vi "Auto Intake Mode.vi"(11 "Intake Commands Cluster":T2={"Intake Commands"=enum."Load", "Intake Mode"=enum."Auto", "Override IR"=FALSE}) -> (0 "Intake States":T1, 1 "Raw Negated Encoder Position":dbl, 2 "Roller Power":dbl, 3 "Angle Power":dbl, 4 "Target Height":dbl, 5 "Encoder Position":dbl, 6 "Rollers Active?":bool)   [LabVIEW 2015]
uses:
  Common Code/Intake Commands Cluster.ctl
  Common Code/Intake Commands.ctl
  Common Code/Intake Mode.ctl
  Common Code/Intake States.ctl
  Robot Global Data.vi
  <vilib>/addons/control/pid/pid.llb/PID (DBL).vi
  <vilib>/addons/control/pid/NI_PID_pid.lvlib
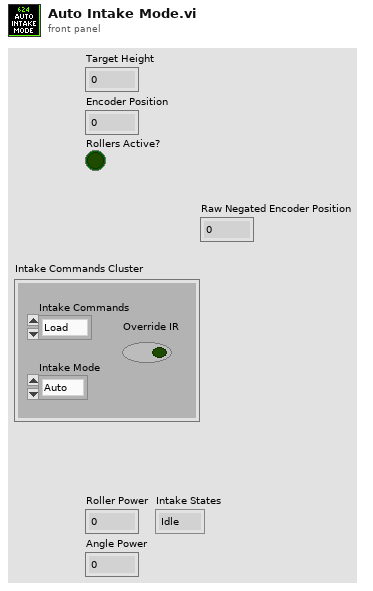
[diagram p1: front panel]
types:
  T1 = typedef "Intake States.ctl" = enum16{"Idle", "Set roller speed", "Move to angle"}
  T2 = typedef "Intake Commands Cluster.ctl" = cluster{"Intake Commands":T3, "Intake Mode":T4, "Override IR":bool}
  T3 = typedef "Intake Commands.ctl" = enum16{"Unload", "Load", "Pull up", "Drop low", "Idle", "Lift Half"}
  T4 = typedef "Intake Mode.ctl" = enum16{"Safe", "Auto", "Manual"}
  T5 = typedef "Dashboard Control Data.ctl" = cluster{"Encoder Control":T6, "Steer PID output":cluster{"output high":dbl, "output low":dbl}, " Steer PID gains":cluster{"proportional gain (Kc)":dbl, "integral time (Ti, min)":dbl, "derivative time (Td, min)":dbl}, "Drivetrain Settings":T7, "Vision Packet":T8, "Info/Command Cluster":T9, "Ball Vision Packet":T10, "Intake Presets":T12, "Intake Encoder Control":T14, "Climb Presets":T15, "Goal Output Range":cluster{"output high":dbl, "output low":dbl}, "Shooter Presets":T16}
  T6 = typedef "Encoder Control.ctl" = cluster{"Right Tick Constant":dbl, "Left Tick Constant":dbl, "Reset?":bool, "Y Dist":cluster{"PID gains":cluster{"proportional gain (Kc)":dbl, "integral time (Ti, min)":dbl, "derivative time (Td, min)":dbl}}, "Y Stop Thresh":dbl, "Y Stop Speed":dbl}
  T7 = typedef "Drivetrain Settings.ctl" = cluster{"Gyro Tolerance":dbl, "Throttle Ramp (ms)":dbl, "Angular rate compensation":bool, "Throttle to Rate Scale":dbl, "Rate compensation gain":dbl, "Kv":dbl, "Ka":dbl, "Feed Forward P":dbl, "Feed Forward D":dbl, "Goal Vision PID gains":cluster{"proportional gain (Kc)":dbl, "integral time (Ti, min)":dbl, "derivative time (Td, min)":dbl}, "Goal Detection Window":dbl}
  T8 = typedef "Goal Vision Packet.ctl" = cluster{"Distance":dbl, "Center X":dbl, "Center Y":dbl, "Found Target?":bool}
  T9 = typedef "Ball Tracking Command Cluster.ctl" = cluster{"Distance to Ball":dbl, "Desired Angle":dbl, "Command":enum16{"Turn to Ball", "Turn to Angle", "Get Distance"}, "Pixels from Center":dbl}
  T10 = typedef "Ball Vision Packet.ctl" = cluster{"Ball Detected?":bool, "Distance to Ball":dbl, "Desired Angle":dbl, "Pixels from Center":dbl, "Tracking mode":T11}
  T11 = typedef "Tracking Mode.ctl" = enum16{"Turn to Ball", "Turn to Angle"}
  T12 = typedef "Intake Presets.ctl" = cluster{"Intake Speed":dbl, "Outake Speed":dbl, "Low Height":dbl, "Half Height":dbl, "Full Height":dbl, "Angle Speed":dbl, "Fast Angle":dbl, "Encoder Scale":dbl, "Load Height":dbl, "Output Range":T13, "Rotation Power Max/Min":dbl, "MaxCurrent":dbl, "Intake Trip Time":dbl, "Idle Height":dbl, "Max Height":dbl, "Reset Encoders?":bool, "PID gains":cluster{"proportional gain (Kc)":dbl, "integral time (Ti, min)":dbl, "derivative time (Td, min)":dbl}}
  T13 = typedef "Drivetrain Output Range.ctl" = cluster{"output high":dbl, "output low":dbl}
  T14 = typedef "IntakeEcoderControl.ctl" = cluster{"Arm Tick Constant":dbl, "Reset?":bool, "Y Dist":cluster{"PID gains":cluster{"proportional gain (Kc)":dbl, "integral time (Ti, min)":dbl, "derivative time (Td, min)":dbl}}, "Y Stop Thresh":dbl, "Y Stop Speed":dbl}
  T15 = typedef "Climb Presets.ctl" = cluster{"Pull Power":dbl, "Unpin Power":dbl, "Time to Hold":dbl}
  T16 = typedef "Shooter Presets.ctl" = cluster{"Batter Shot":T17, "Deep Middle Shot":T17, "Manual Shot":T17, "Left Ticks Per Rotation":dbl, "Right Ticks Per Rotation":dbl, "Low Bar Shot":T17, "Shooter RPM Tolerance":dbl, "IIR Filter Power":dbl, "Trigger Power":dbl, "Fire from Load Delay":i32, "Angle Pot M":dbl, "Angle Pot B":dbl, "Shooter Length":dbl, "String Pot Dist":dbl, "Angle PID gains":cluster{"proportional gain (Kc)":dbl, "integral time (Ti, min)":dbl, "derivative time (Td, min)":dbl}, "Angle Motor Output":cluster{"output high":dbl, "output low":dbl}, "Shooter Angle Tolerance":dbl, "Vision Shoot x^2":dbl, "Vision Shoot x":dbl, "Dist from Axis Cam to Pivot":dbl, "High Goal Center Height":dbl, "Feed Forward Max Accel":dbl, "Feed Forward Kv":dbl, "Backwards Trigger":dbl, "Shot Finish Delay (ms)":dbl, "Angle Max Current":dbl, "Angle Current Trip Time":dbl, "Shooter Intake Angle":dbl, "Vision Shoot c":dbl, "Reset?":bool, "Servo Release Delay":dbl, "Servo Idle Angle":i32, "Servo Hold Angle":i32, "Angle Pot x^2":dbl, "Angle Pot x":dbl, "Angle Pot c":dbl}
  T17 = typedef "Shot Presets.ctl" = cluster{"Left Wheel RPM":dbl, "Right Wheel RPM":dbl, "Angle":dbl}
  T18 = cluster{"proportional gain (Kc)":dbl, "integral time (Ti, min)":dbl, "derivative time (Td, min)":dbl}
  T19 = typedef "WPI_MotorControlDeviceRef.ctl" = cluster{"DeviceStatus":errorcluster, "Type":T20, "PWM":cluster{"PWM Channel":T21, "DeadBand":T22}, "CAN":cluster{"Device Number":u8, "Control Mode":T23, "Semaphore":T24, "Max Vout":dbl, "TalonSRX Control Mode":T25}, "Invert":bool}
  T20 = typedef "WPI_MotorControlType.ctl" = enum16{"PWM", "CAN", "CANTalonSRX"}
  T21 = typedef "FPGA_DIOPWMChannel.ctl" = enum8{"PWM 0", "PWM 1", "PWM 2", "PWM 3", "PWM 4", "PWM 5", "PWM 6", "PWM 7", "PWM 8", "PWM 9", "PWM MXP 0", "PWM MXP 1", "PWM MXP 2", "PWM MXP 3", "PWM MXP 4", "PWM MXP 5", "PWM MXP 6", "PWM MXP 7", "PWM MXP 8", "PWM MXP 9", "Invalid"}
  T22 = typedef "WPI_PWMDeadband.ctl" = cluster{"Name":string, "maxPositivePwm":i32, "minPositivePwm":i32, "centerPwm":i32, "maxNegativePwm":i32, "minNegativePwm":i32, "angularRange":u16}
  T23 = typedef "WPI_CANJaguar_ControlMode.ctl" = enum8{"Percent VBus", "Current", "Speed", "Position", "Voltage"}
  T24 = typedef "Semaphore RefNum" = refnum<k1>
  T25 = typedef "WPI_CANTalonSRX_APIControlMode.ctl" = enum8{"Percent VBus", "Speed", "Position", "Slave", "Unchanged / Invalid", "Voltage Compensation", "Current", "Motion Profile"}
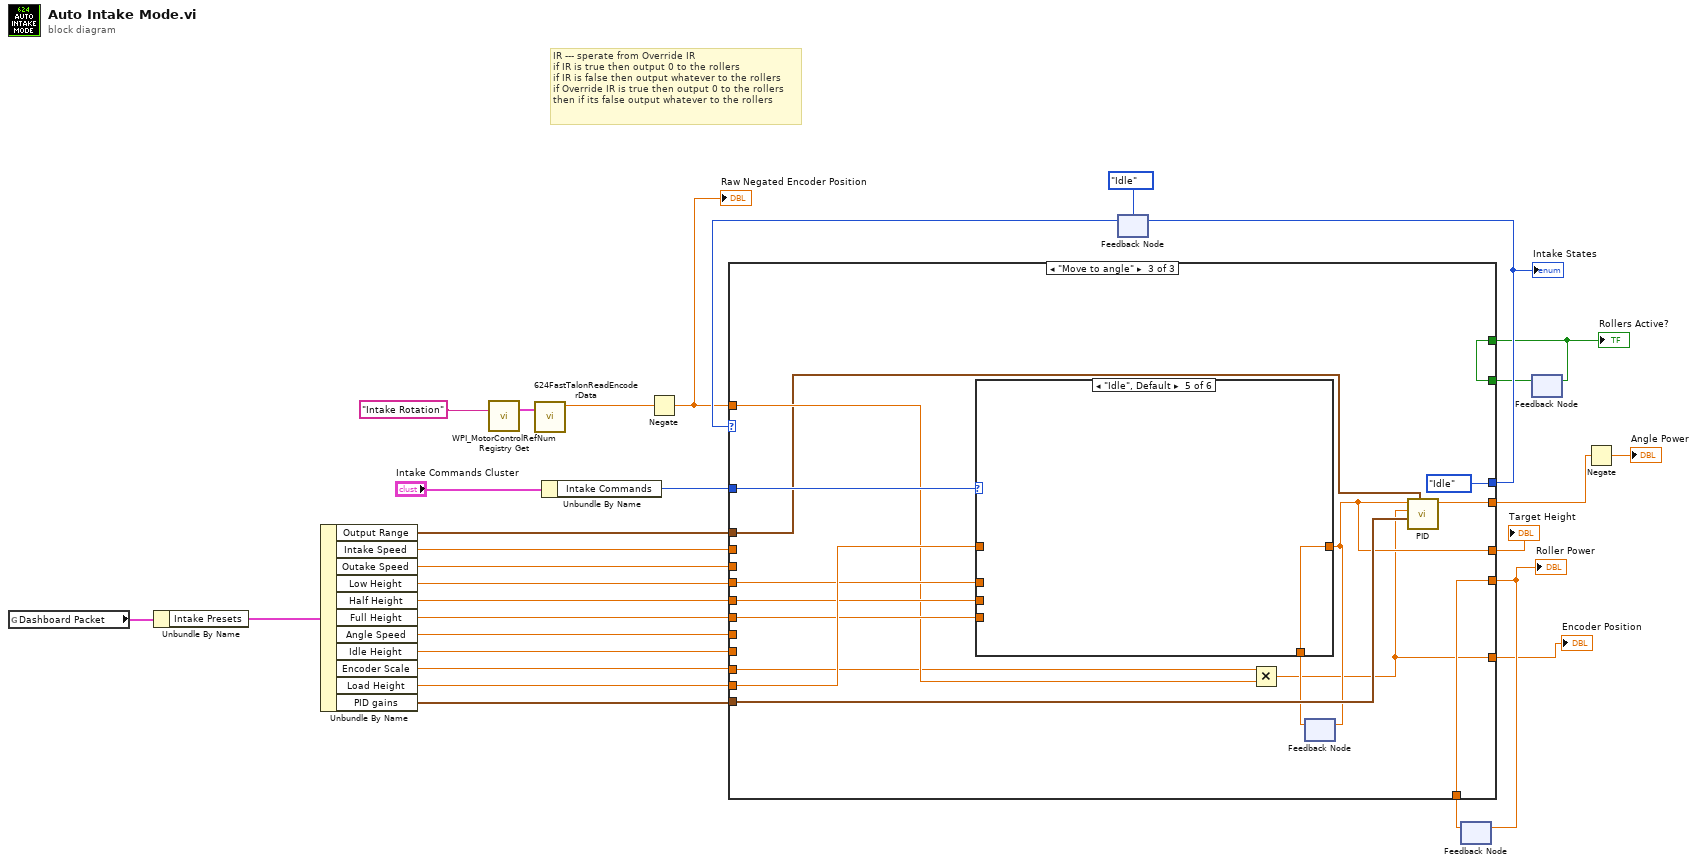
[diagram p0: block diagram]
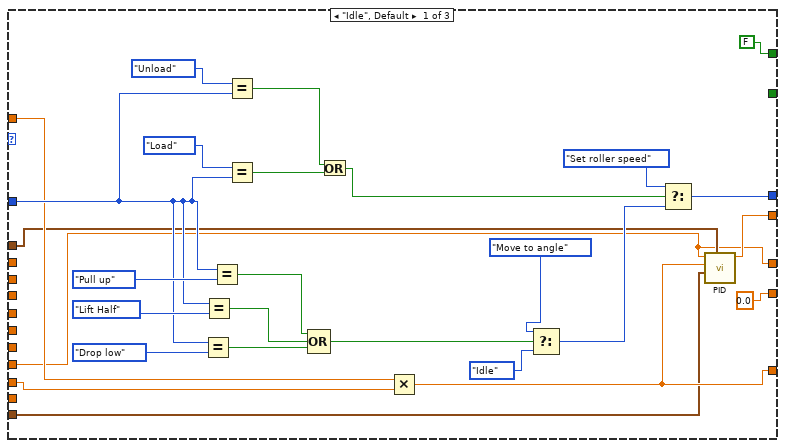
[diagram p2: hidden frame]
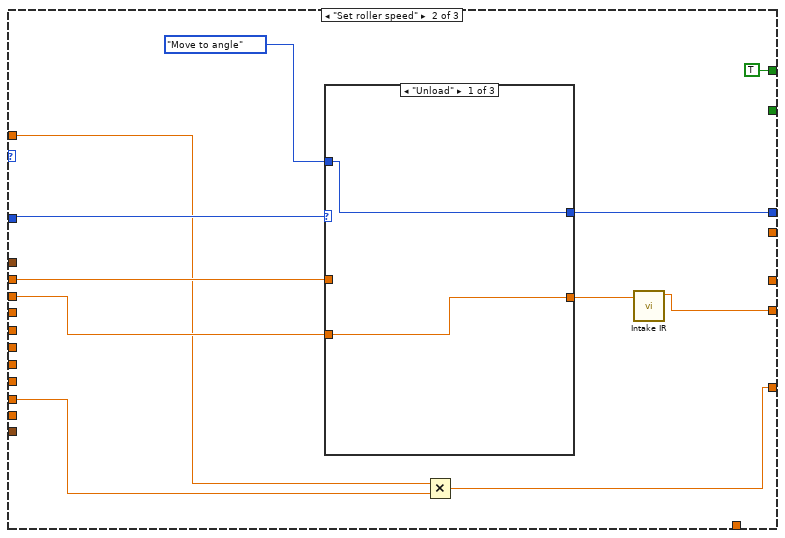
[diagram p3: hidden frame]
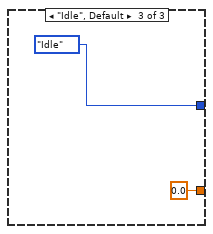
[diagram p5: hidden frame]
diagram:
  # "IR --- sperate from Override IR \nif IR is true then output 0 to the rollers\nif IR is false then output whatever to the rollers\nif Override IR is true then output 0 to the rollers\nthen if its false output whatever to the rollers"
  n1 = global read "Robot Global Data.vi" "Dashboard Packet"() -> (w1:T5)
  n2 = Unbundle By Name(w1) -> ("Intake Presets"=w2:T12)
  n3 = Unbundle By Name(w2) -> ("Output Range"=w13:T13, "Intake Speed"=w12:dbl, "Outake Speed"=w11:dbl, "Low Height"=w10:dbl, "Half Height"=w9:dbl, "Full Height"=w8:dbl, "Angle Speed"=w7:dbl, "Idle Height"=w6:dbl, "Encoder Scale"=w5:dbl, "Load Height"=w4:dbl, "PID gains"=w3:T18)
  n4 = call <vilib>:"WPI_MotorControlRefNum Registry Get.vi"("refnum name"="Intake Rotation") -> ("MotorControlDevRef"=w22:T19)  [unwired: 9 in, 1 out]
  n5 = call "624FastTalonReadEncoderData.vi"("CAN Talon SRX Ref"=w22) -> ("Encoder Position"=w19:dbl)  [unwired: 5 in, 5 out]
  n6 = Unbundle By Name("Intake Commands Cluster") -> ("Intake Commands"=w27:T3)
  n7 = Negate(x=w19) -> (-x=w18:dbl)
  "Raw Negated Encoder Position" <- w18
  n8 = feedback #1(Intake_States."Idle") -> (w29:T1)
  n9 = feedback #2() -> (w24:dbl)  [unwired: 1 in]
  n10 = feedback #3() -> (w16:bool)  [unwired: 1 in]
  n11 = case shown="\"Move to angle\"" w29 {
    tunnel: w27 -> [w43 w68 w90]
    tunnel: [w47 w66 Intake_States."Idle"] -> w26
    tunnel: w13 -> [w34 _ w79]
    tunnel: w11 -> [_ w64 _]
    tunnel: w8 -> [_ _ w85]
    tunnel: w12 -> [_ w65 _]
    tunnel: w9 -> [_ _ w87]
    tunnel: w7 -> [_ _ _]
    tunnel: w10 -> [_ _ w86]
    tunnel: [0.0 ("Intake Speed") w59 w89] -> w25
    tunnel: w24 -> [_ _ w89]
    tunnel: w4 -> [_ _ w88]
    tunnel: [w33 _ w83] -> w14
    tunnel: w18 -> [w37 w63 w82]
    tunnel: w5 -> [w38 w62 w81]
    tunnel: w3 -> [w35 _ w80]
    tunnel: w6 -> [w32 _ _]
    tunnel: [w32 _ w78] -> w21
    tunnel: [w36 w61 w76] -> w20
    tunnel: [FALSE TRUE w75] -> w17
    tunnel: w16 -> [_ _ w75]
    frame "Idle", Default {
      n12 = Equal?(x=w43, y=Intake_Commands."Drop low" ("Intake Commands")) -> (x = y?=w49:bool)
      n13 = Equal?(x=w43, y=Intake_Commands."Lift Half" ("Intake Commands")) -> (x = y?=w50:bool)
      n14 = Equal?(x=w43, y=Intake_Commands."Pull up" ("Intake Commands")) -> (x = y?=w54:bool)
      n15 = Equal?(x=Intake_Commands."Unload" ("Intake Commands"), y=w43) -> (x = y?=w42:bool)
      n16 = Equal?(x=Intake_Commands."Load" ("Intake Commands"), y=w43) -> (x = y?=w41:bool)
      n17 = Compound Arithmetic op=OR(w54, w50, w49) -> (w53:bool)
      n18 = Or(x=w42, y=w41) -> (x .or. y?=w40:bool)
      n19 = Multiply(x=w37, y=w38) -> (x*y=w36:dbl)
      n20 = Select(t=Intake_States."Move to angle", s=w53, f=Intake_States."Idle") -> (s? t:f=w48:T1)
      n21 = Select(t=Intake_States."Set roller speed", s=w40, f=w48) -> (s? t:f=w47:T1)
      n22 = call-poly <vilib>:"PID.vi"("output range"=w34, "PID gains"=w35, "process variable"=w36, "setpoint"=w32) -> ("output"=w33:dbl)  [unwired: 6 in, 1 out]
    }
    frame "Set roller speed" {
      n23 = case shown="\"Unload\"" w68 {
        tunnel: Intake_States."Move to angle" -> [w70 w72 _]
        tunnel: [w70 w72 Intake_States."Idle"] -> w66
        tunnel: w65 -> [_ w71 _]
        tunnel: [w69 w71 0.0 ("Intake Speed")] -> w58
        tunnel: w64 -> [w69 _ _]
        frame "Unload" {
        }
        frame "Load" {
        }
        frame "Idle", Default {
        }
      }
      n24 = Multiply(x=w63, y=w62) -> (x*y=w61:dbl)
      n25 = call "Intake IR.vi"("Speed"=w58) -> ("Speeeeeeed"=w59:dbl)  [unwired: 10 in]
    }
    frame "Move to angle" {
      n26 = Multiply(x=w81, y=w82) -> (x*y=w76:dbl)
      n27 = feedback #4() -> (w77:dbl)  [unwired: 1 in]
      n28 = case shown="\"Idle\", Default" w90 {
        tunnel: w88 -> [w91 w92 _ _ _ _]
        tunnel: [w91 w92 w93 w94 w95 w96] -> w78
        tunnel: w87 -> [_ _ _ _ _ w96]
        tunnel: w86 -> [_ _ _ w94 _ _]
        tunnel: w85 -> [_ _ w93 _ _ _]
        tunnel: w77 -> [_ _ _ _ w95 _]
        frame "Unload" {
        }
        frame "Load" {
        }
        frame "Pull up" {
        }
        frame "Drop low" {
        }
        frame "Idle", Default {
        }
        frame "Lift Half" {
        }
      }
      n29 = feedback-in #4(w78) -> ()
      n30 = call-poly <vilib>:"PID.vi"("output range"=w79, "PID gains"=w80, "process variable"=w76, "setpoint"=w78) -> ("output"=w83:dbl)  [unwired: 6 in, 1 out]
    }
  }
  "Roller Power" <- w25
  "Intake States" <- w26
  "Target Height" <- w21
  "Encoder Position" <- w20
  "Rollers Active?" <- w17
  n31 = feedback-in #1(w26) -> ()
  n32 = feedback-in #2(w25) -> ()
  n33 = feedback-in #3(w17) -> ()
  n34 = Negate(x=w14) -> (-x=→"Angle Power":dbl)
